vi "Find OOB Server Ports.vi"(8 "error in":errorcluster) -> (3 "Ports":u16[](array[numeric]))   [LabVIEW 2025]
panel:
  out "return code":i32
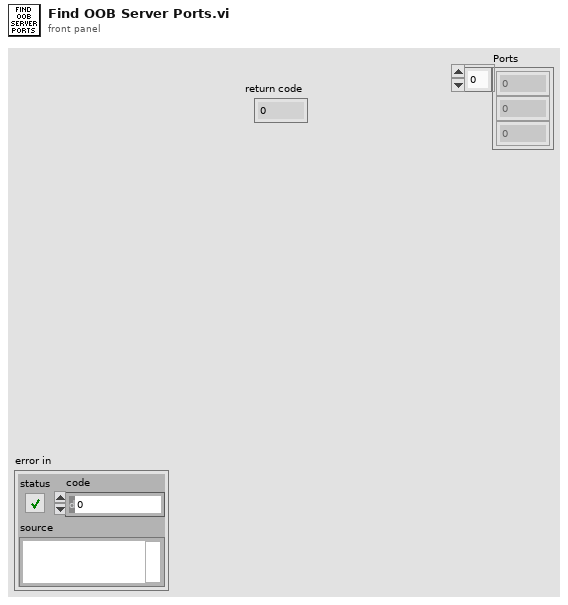
[diagram p1: front panel]
types:
  T1 = cluster{"Protocol":enum16{"invalid", "tcp", "udp", "icmp", "ip", "tcpv6", "udpv6", "icmpv6", "ipv6"}, "LocalIP":string, "LocalPort":u16, "ForeignIP":string, "ForeignPort":u16, "State":enum8{"UNKNOWN", "LISTEN", "ESTABLISHED", "SYN_SENT", "SYN_RECV", "LAST_ACK", "CLOSE_WAIT", "TIME_WAIT", "CLOSED", "CLOSING", "FIN_WAIT1", "FIN_WAIT2"}, "PID":u16}[]
  T2 = enum8{"UNKNOWN", "LISTEN", "ESTABLISHED", "SYN_SENT", "SYN_RECV", "LAST_ACK", "CLOSE_WAIT", "TIME_WAIT", "CLOSED", "CLOSING", "FIN_WAIT1", "FIN_WAIT2"}
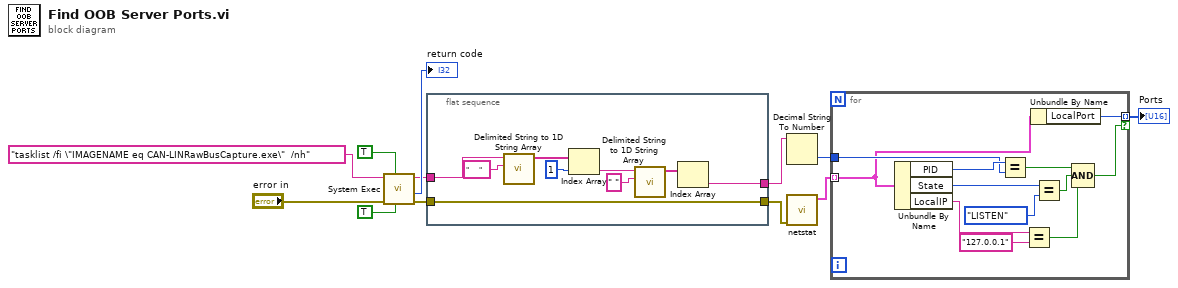
[diagram p0: block diagram]
diagram:
  n1 = call <vilib>:"System Exec.vi"("run minimized? (F)"=TRUE, "wait until completion? (T)"=TRUE, "error in (no error)"="error in", "command line"="tasklist /fi \"IMAGENAME eq CAN-LINRawBusCapture.exe\"  /nh") -> ("error out"=w7:errorcluster, "return code"=→"return code":i32, "standard output"=w5:string)  [unwired: 4 in, 1 out]
  n2 = flat-sequence {
    tunnel: w5 -> [w21]
    tunnel: [w14] -> w6
    tunnel: w7 -> [w13]
    tunnel: [w13] -> w2
    frame #0 {
      n3 = call <vilib>:"Delimited String to 1D String Array.vi"("delimiter"="     ", "delimited string"=w21) -> ("string array"=w19:string[])  [unwired: 9 in]
      n4 = Index Array(array=w19, index=1) -> (element=w17:string)
      n5 = call <vilib>:"Delimited String to 1D String Array.vi"("delimiter"=" ", "delimited string"=w17) -> ("string array"=w15:string[])  [unwired: 9 in]
      n6 = Index Array(array=w15) -> (element=w14:string)  [unwired: 1 in]
    }
  }
  n7 = Decimal String To Number(string=w6) -> (number=w4:i32)  [unwired: 2 in, 1 out]
  n8 = call "netstat.vi"("error in (no error)"=w2) -> ("netstat"=w3:T1)  [unwired: 9 in, 1 out]
  n9 = for {
    tunnel: w3 -> [w24] mode=indexing
    tunnel: w4 -> [w32]
    tunnel: [w23] -> w1 mode=indexing if=w22
    n10 = Unbundle By Name(w24) -> ("PID"=w33:u16, "State"=w30:T2, "LocalIP"=w27:string)
    n11 = Equal?(x=w33, y=w32) -> (x = y?=w31:bool)
    n12 = Equal?(x=w27, y="127.0.0.1") -> (x = y?=w25:bool)
    n13 = Unbundle By Name(w24) -> ("LocalPort"=w23:u16)
    n14 = Equal?(x=w30, y=T2."LISTEN") -> (x = y?=w28:bool)
    n15 = Compound Arithmetic op=AND(w31, w28, w25) -> (w22:bool)
  }
  "Ports" <- w1
